vi "RQST Lookup Table Initialize.vi"(8 "error in (no error)":errorcluster) -> (0 "error out":errorcluster {"code" min=0 max=0}, 3 "Rqst LUT":T1)   [LabVIEW 2015, in "J1939 Addon Engine.lvlib"]
uses:
  J1939 Addon Engine.lvlib
  Types/RQST Lookup Table Reference.ctl
  Types/RQST Lookup Table Action.ctl
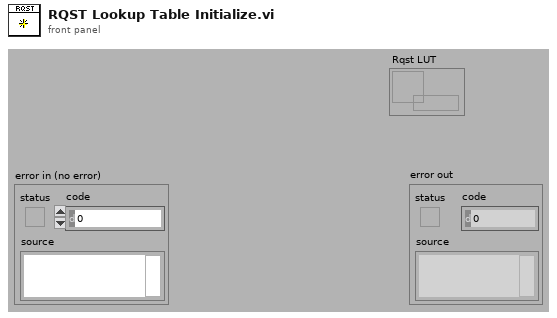
[diagram p1: front panel]
types:
  T1 = typedef "J1939 Addon Engine.lvlib/RQST Lookup Table Reference.ctl" = refnum<data-value>
  T2 = typedef "J1939 Addon Engine.lvlib/RQST Lookup Table Action.ctl" = enum16{"Initialize", "Add", "Get", "Remove"}
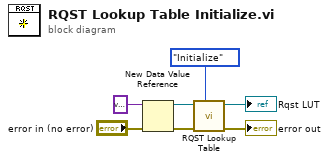
[diagram p0: block diagram]
diagram:
  n1 = New Data Value Reference(data value=variant ("variant"), error in="error in (no error)") -> (data value reference=w4:refnum<data-value>, error out=w5:errorcluster)
  n2 = call "RQST Lookup Table.vi"("Action"=RQST_Lookup_Table_Action."Initialize", "error in (no error)"=w5, "Rqst LUT"=w4) -> ("error out"=→"error out":errorcluster, "Rqst LUT out"=→"Rqst LUT":T1)  [unwired: 5 in, 2 out]
